vi "作业2（第二题）.vi"() -> ()   [LabVIEW 2017]
panel:
  out "平均值":dbl
  out "求和":dbl
  in  "C":dbl
  in  "B":dbl
  in  "A":dbl
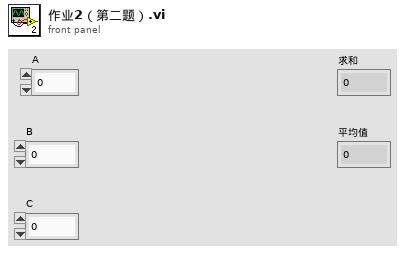
[diagram p1: front panel]
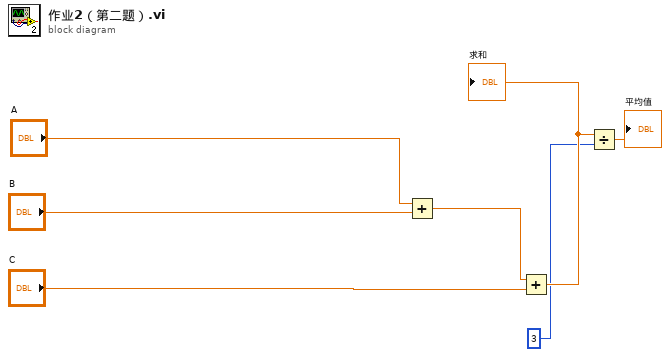
[diagram p0: block diagram]
diagram:
  n1 = Add(x="A", y="B") -> (x+y=w4:dbl)
  n2 = Add(x=w4, y="C") -> (x+y=w3:dbl)
  "求和" <- w3
  n3 = Divide(x=w3, y=3) -> (x/y=→"平均值":dbl)
